vi "GPS.vi"() -> ()   [LabVIEW 2015]
uses:
  <vilib>/MakerHub/LINX/Public/Utilities/Open Serial.vi
  <vilib>/MakerHub/LINX/LMH-LINX.lvlib
  <vilib>/MakerHub/LINX/Public/Sensors/Pmods/GPS/PmodGPS.lvlib
panel:
  out "GPS Data":T1
  in  "GPS Channel":T2(ring)=enum."RX3 - Pin15"
  in  "Serial Port":refnum<visa-resource-name>="N/A"
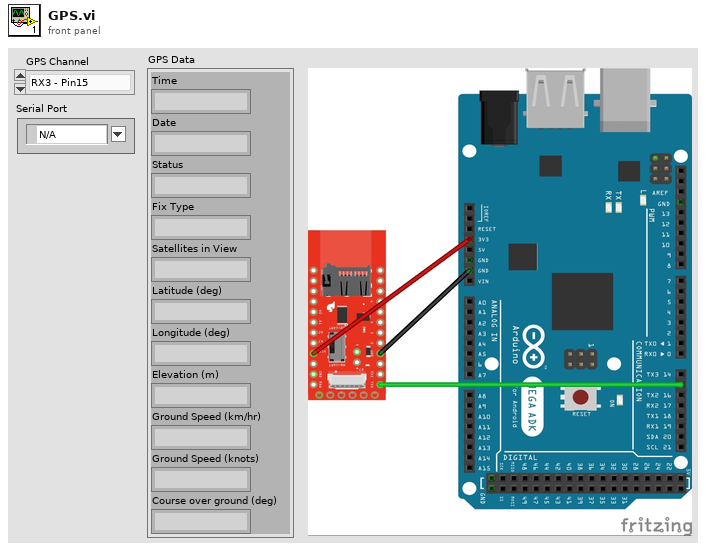
[diagram p1: front panel]
types:
  T1 = cluster{"Time":string, "Date":string, "Status":string, "Fix Type":string, "Satellites in View":string, "Latitude (deg)":string, "Longitude (deg)":string, "Elevation (m)":string, "Ground Speed (km/hr)":string, "Ground Speed (knots)":string, "Course over ground (deg)":string}
  T2 = enum16{"RX0 - Pin0", "RX1 - Pin17", "RX2 - Pin19", "RX3 - Pin15"}
  T3 = typedef "LMH-LINX.lvlib/LINX Ref.ctl" = cluster{"IO":T4, "Interface":T5, "LINX Device Config":T6}
  T4 = typedef "LMH-LINX.lvlib/Platform.ctl" = enum16{"Remote", "Local"}
  T5 = typedef "LMH-LINX.lvlib/Interface.ctl" = enum16{"Serial", "TCP"}
  T6 = typedef "LMH-LINX.lvlib/Device.lvlib/LINX Device Config.ctl" = cluster{"Interface":T5, "COM Port":refnum<visa-resource-name>, "TCP Configuration":T7, "Device Family":u8, "Device ID":u8, "Device Name":string, "TCP Ref":refnum<k5>, "Channels":T8}
  T7 = typedef "LMH-LINX.lvlib/Device.lvlib/TCP Config.ctl" = cluster{"IP Address":string, "Port":u16}
  T8 = typedef "LMH-LINX.lvlib/Channels.ctl" = cluster{"DI":u8[], "DO":u8[], "AI":u8[], "AO":u8[], "PWM":u8[], "QE":u8[], "UART":u8[], "I2C 2":u8[], "SPI":u8[], "CAN":u8[], "Servo":u8[], "AI Ref (V)":dbl, "AI Resolution (Bits)":u8, "AO Ref (V)":dbl, "AO Resolution (Bits)":u8}
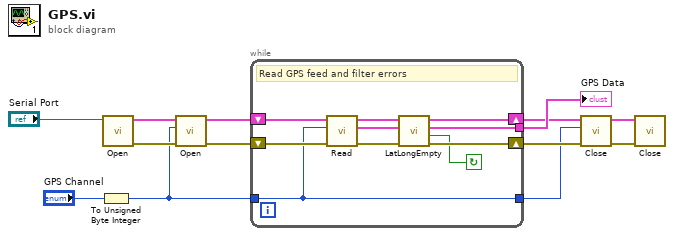
[diagram p0: block diagram]
diagram:
  n1 = To Unsigned Byte Integer(number="GPS Channel") -> (unsigned 8bit integer=w2:u8)
  n2 = call-poly <vilib>:"Open.vi"("Serial Port"="Serial Port") -> ("Error Out"=w10:errorcluster, "LINX Resource"=w11:T3)  [unwired: 8 in, 1 out]
  n3 = call <vilib>:"Open.vi"("Error In"=w10, "UART Channel (0)"=w2, "LINX Ref"=w11) -> ("Error Out"=w8:errorcluster, "LINX Resource"=w9:T3)  [unwired: 7 in]
  n4 = while {
    shift-right: [w17] -> w6
    shift-left: w8 -> [w22]
    shift-right: [w20] -> w7
    shift-left: w9 -> [w23]
    tunnel: [w16] -> w13
    tunnel: w2 -> [w14]
    tunnel: [w14] -> w1
    stop <- w15 continue-if-true
    # "Read GPS feed and filter errors"
    n5 = call <vilib>:"Read.vi"("Error In"=w22, "UART Channel (0)"=w14, "LINX Resource"=w23) -> ("Error Out"=w18:errorcluster, "GPS Data"=w19:T1, "LINX Resource"=w21:T3)  [unwired: 6 in]
    n6 = call "LatLongEmpty.vi"("error (in)"=w18, "GPS Data"=w19, "LINX Resource"=w21) -> ("error (out)"=w17:errorcluster, "Empty or not in range?"=w15:bool, "GPS Data"=w16:T1, "LINX Resource"=w20:T3)  [unwired: 5 in]
  }
  "GPS Data" <- w13
  n7 = call <vilib>:"Close.vi"("error in (no error)"=w6, "UART Channel (0)"=w1, "LINX Resource"=w7) -> ("error out"=w4:errorcluster, "LINX Resource out"=w5:T3)  [unwired: 7 in]
  n8 = call <vilib>:"Close.vi"("Error In"=w4, "LINX Resource"=w5) -> ()  [unwired: 9 in, 1 out]
